vi "Machine Read_Write Test.vi"(0 "VISA resource name":refnum<visa-resource-name>="COM1", 1 "baud rate":u32=9600, 2 "data bits":u16=8 min=5 max=8 step=1, 3 "parity":u16(ring) items=["None", "Odd", "Even", "Mark", "Space"], 4 "stop bits":u16(ring)=10 items=["1.0"=10, "1.5"=15, "2.0"=20], 5 "write":bool, 7 "flow control":u16(ring) items=["None"=0, "XON/XOFF"=1, "RTS/CTS"=2, "DTR/DSR"=4], 8 "string to write":string="*IDN?") -> (9 "read string":string)   [LabVIEW 2016]
doc: "The Basic Serial Read and Write example performs a Serial Port Read, a Serial Port Write, or a combination of these actions. The user selects the actions (read or write) on the front panel. If both are selected, the VI will write the data first, read data, and then close the VISA session that is opened to the port. This VI will wait until the specified number of bytes is received at the port. Only the number of bytes specified will be read.\n\nINSTRUCTIONS:\n1) Select the serial resource and configuration parameters (baud rate, data bits, parity, stop bits, flow control).\n2) Select the operations to be performed. \n3) Connect the serial port to your device. If no device is available, perform a loopback test by doing one of the following. Short pins 2 and 3 on a RS-232 cable or short pin 4 to pin 8 and pin 5 to pin 9 on a RS-485/422 cable. \n4) Run the VI to see the data read. (The \"read string\" will match the \"string to write\" if a loopback test was performed.)\n\nNote: The parameters set for the serial port must match the parameters of the connected instrument or device. In this example, the bytes to read parameter specifies the number of bytes that the serial port reads. If there were more bytes at the port than the number specified in bytes to read, those bytes would not be read. Also, if you specify to read more bytes than the number of bytes actually read, you might receive a timeout error message.\n\nOn the block diagram, the Configure Serial Port VI sets the configuration parameters. The front panel displays the controls used to configure the basic parameters, such as baud rate, data bits, and parity. Constants configure the other parameters the user probably does not need set. After the VISA Configure Serial Port VI opens the VISA session and configures the port, the VI passes the VISA resource name to other VIs that perform operations on that VISA resource. The VISA Write function sends a command to the serial device and the VISA Read function returns data based on the command. The VISA Close function then closes the reference to the serial device. It is important to close the reference; otherwise communication through with that port through protocols other than VISA might not be possible."
uses:
  <vilib>/Instr/_visa.llb/VISA Configure Serial Port (Instr).vi
panel:
  in  "stop":bool
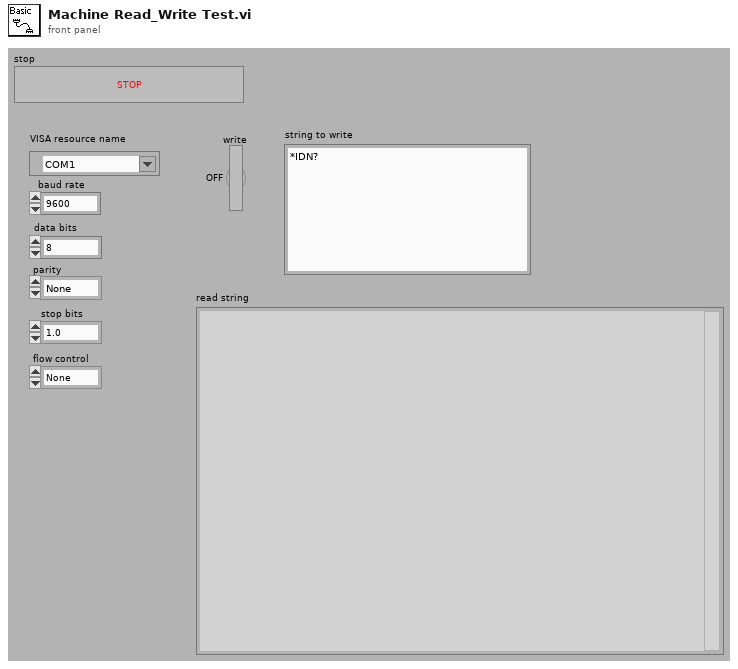
[diagram p1: front panel]
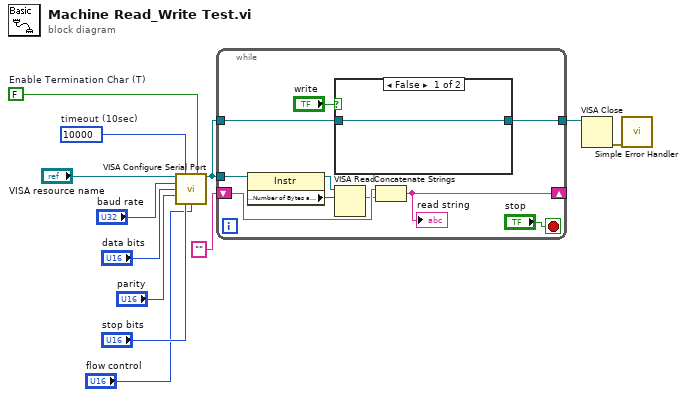
[diagram p0: block diagram]
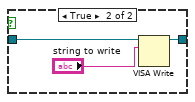
[diagram p2: hidden frame]
diagram:
  w7 = FALSE  # Enable Termination Char (T)
  w8 = u32 10000  # timeout (10sec)
  n1 = call-poly "VISA Configure Serial Port"("VISA resource name"="VISA resource name", "timeout (10sec)"=w8, "Enable Termination\nChar (T)"=w7, "baud rate (9600)"="baud rate", "data bits (8)"="data bits", "parity (0:none)"="parity", "stop bits (10: 1 bit)"="stop bits", "flow control (0:none)"="flow control") -> ("VISA resource name out"=w2:refnum<visa-resource-name>)  [unwired: 6 in, 1 out]
  n2 = while {
    tunnel: w2 -> [w22]
    shift-right: [w17] -> _
    shift-left: "" -> [w19]
    tunnel: w2 -> [w14]
    tunnel: [w13] -> w1
    stop <- "stop" stop-if-true
    n3 = property class="Instr"(reference=w22) -> (reference out=w20:refnum<visa-resource-name>, "Serial Settings:Number of Bytes at Serial Port"=w21:u32)  [unwired: 1 in, 1 out]
    n4 = case shown="False" "write" {
      tunnel: w14 -> [w23 w25]
      tunnel: [w23 w24] -> w13
      frame False {
      }
      frame True {
        n5 = VISA Write(VISA resource name=w25, write buffer="string to write") -> (VISA resource name out=w24:refnum<visa-resource-name>)  [unwired: 1 in, 2 out]
      }
    }
    n6 = VISA Read(VISA resource name=w20, byte count=w21) -> (read buffer=w18:string)  [unwired: 1 in, 3 out]
    n7 = Concatenate Strings(w19, w18) -> (w17:string)
    "read string" <- w17
  }
  n8 = VISA Close(VISA resource name=w1) -> (error out=w10:errorcluster)  [unwired: 1 in]
  n9 = call <vilib>:"Simple Error Handler.vi"("error in (no error)"=w10) -> ()  [unwired: 4 in, 5 out]
